vi "Get Scanner (Continuous).vi"(8 "error in (no error)":errorcluster, 11 "Lakeshore Gaussmeter in":refnum<class "Lakeshore Gaussmeter.lvclass">) -> (0 "error out":errorcluster, 2 "Magnetic Field Lakeshore Continuous.lvclass out":refnum<class "Magnetic Field Lakeshore Continuous.lvclass">)   [LabVIEW 2023, in "Lakeshore Gaussmeter.lvclass"]
uses:
  Lakeshore Gaussmeter.lvclass
  Scanners/Magnetic Field Lakeshore Continuous/Magnetic Field Lakeshore Continuous.lvclass
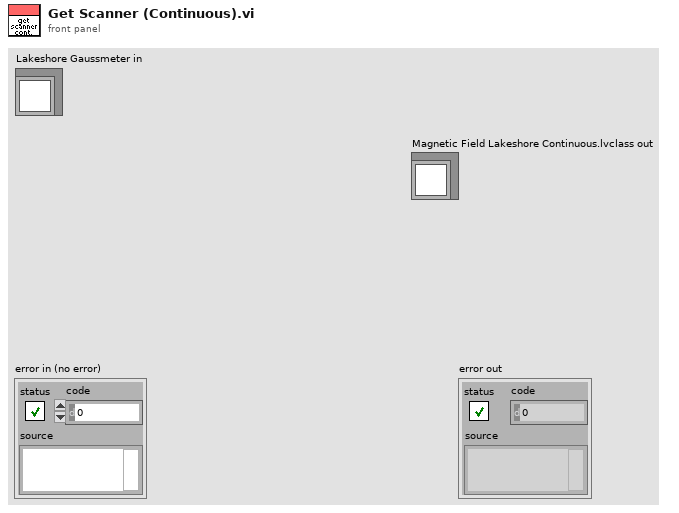
[diagram p1: front panel]
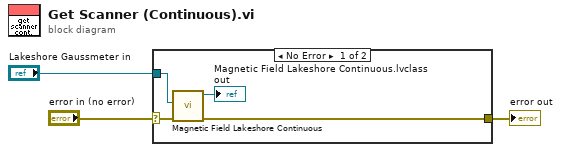
[diagram p0: block diagram]
diagram:
  n1 = case shown="No Error" "error in (no error)" {
    selector: "error in (no error)" -> [w5 w8]
    tunnel: [w4 w8] -> w3
    tunnel: "Lakeshore Gaussmeter in" -> [w6 _]
    frame No Error {
      n2 = call "Magnetic Field Lakeshore Continuous.vi"("error in (no error)"=w5, "Lakeshore Gaussmeter.lvclass"=w6) -> ("error out"=w4:errorcluster, "Magnetic Field Lakeshore Continuous.lvclass out"=→"Magnetic Field Lakeshore Continuous.lvclass out":refnum<class "Magnetic Field Lakeshore Continuous.lvclass">)  [unwired: 8 in]
    }
    frame Error {
    }
  }
  "error out" <- w3
